vi "AO Repeat（Host）.vi"() -> ()   [LabVIEW 2019]
uses:
  <vilib>/FPGAPlugInAG/ELVIS III/niLvFpga_Open_ELVIS III.vi
  <vilib>/rvi/interface/common/dynamic/niFpgaDynamicAddResources.vi
  <vilib>/rvi/interface/common/niFpgaWaitOnOcc.vi
  <vilib>/Utility/error.llb/Error Cluster From Error Code.vi
  <vilib>/rvi/errors/niLvFpgaAdjustHostInterfaceError.vi
  <vilib>/FPGAPlugInAG/Dynamic/niLvFpga_Run_Dynamic.vi
  <vilib>/FPGAPlugInAG/Dynamic/niLvFpga_Abort_Dynamic.vi
  <vilib>/FPGAPlugInAG/Dynamic/niLvFpga_Close_Dynamic.vi
  <vilib>/rvi/interface/nirviOpenFPGA/nirviOpenFPGA.xnode
  FPGA Bitfiles/aiofpga_FPGATarget_AORepeat_+fFBwWQeRIY.lvbitx
  AO Repeat.vi
  <vilib>/rvi/interface/nirviMethod/nirviMethod.xnode
  <vilib>/rvi/interface/nirviReadWriteControl/nirviReadWriteControl.xnode
  <vilib>/rvi/interface/nirviCloseFPGA/nirviCloseFPGA.xnode
  <vilib>/FPGAPlugInAG/Dynamic/niLvFpga_ConfigureFifo_Dynamic.vi
  <vilib>/rvi/errors/niLvFpgaMergeErrorWithErrorCode.vi
  NiFpgaLv.dll
  <vilib>/rvi/interface/Simulation/niFpgaSimulationCallBeginRW.vi
  <vilib>/FPGAPlugInAG/Dynamic/niLvFpga_WriteFifo_Dynamic.vi
panel:
  in  "停止":bool
  in  "B1 采样率 [Hz] 4":dbl=10000.0 min=1000.0 max=1600000.0
  in  "B0 采样率 [Hz] 3":dbl=10000.0 min=1000.0 max=1600000.0
  in  "A1 采样率 [Hz] 2":dbl=10000.0 min=1000.0 max=1600000.0
  in  "A0 采样率 [Hz]":dbl=10000.0 min=1000.0 max=1600000.0
  in  "最大采样点数":dbl=10000.0
  in  "采样点数":u32=1000
  in  "B1 信号频率":dbl=400.0
  in  "B0 信号频率":dbl=200.0
  in  "A1 信号频率":dbl=100.0
  in  "A0 信号频率":dbl=10.0
  out "B1":dbl[](graph)
  out "B0":dbl[](graph)
  out "A1":dbl[](graph)
  out "A0":dbl[](graph)
  in  "Enable":bool[](array[boolean])=[TRUE, FALSE, TRUE, TRUE]
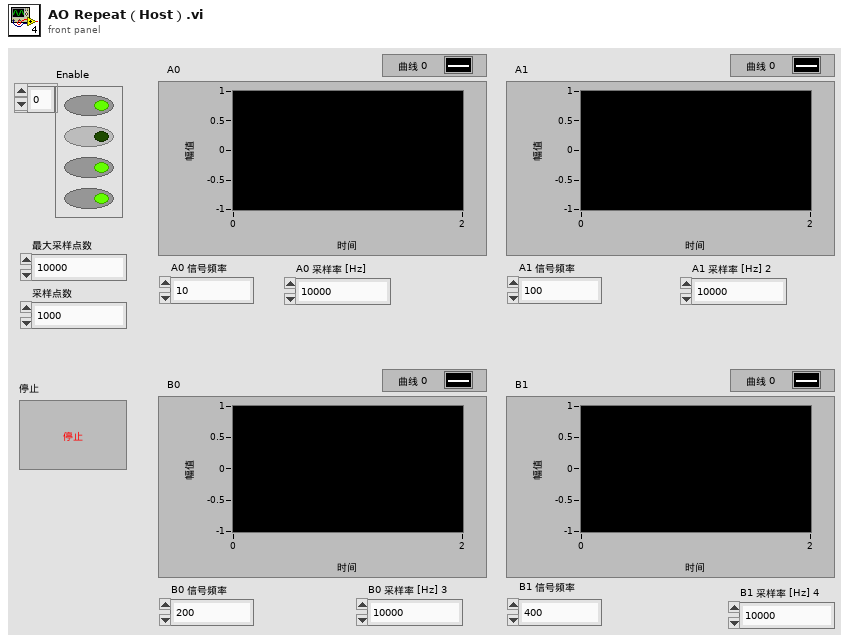
[diagram p1: front panel]
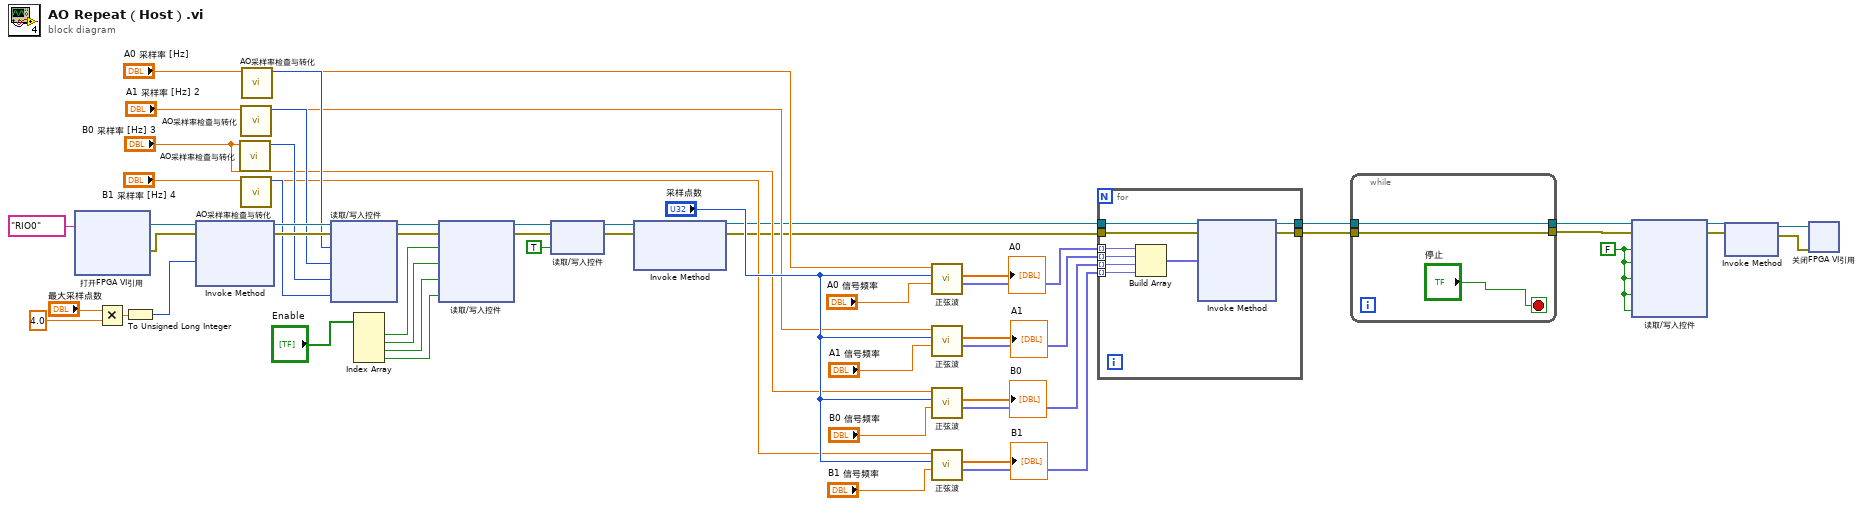
[diagram p0: block diagram]
diagram:
  w7 = FALSE ("开始")
  n1 = xnode "打开FPGA VI引用"("资源名称"=tag "RIO0") -> ("FPGA VI引用输出"=w51:refnum<k20>, "错误输出"=w52:errorcluster)  [unwired: 1 in]
  n2 = Multiply(x="最大采样点数", y=4.0) -> (x*y=w48:dbl)
  n3 = To Unsigned Long Integer(number=w48) -> (unsigned 32bit integer=w47:u32)
  n4 = xnode "Invoke Method"("FPGA VI引用输入"=w51, "错误输入"=w52, "请求的深度"=w47) -> ("FPGA VI引用输出"=w46:refnum<k20>, "错误输出"=w45:errorcluster)  [unwired: 1 out]
  n5 = call "AO采样率检查与转化.vi"("AO FIFO Sample Rate"="B0 采样率 [Hz] 3") -> ("Count (tick/s)"=w41:u32)  [unwired: 9 in, 1 out]
  n6 = call "AO采样率检查与转化.vi"("AO FIFO Sample Rate"="A1 采样率 [Hz] 2") -> ("Count (tick/s)"=w42:u32)  [unwired: 9 in, 1 out]
  n7 = call "AO采样率检查与转化.vi"("AO FIFO Sample Rate"="B1 采样率 [Hz] 4") -> ("Count (tick/s)"=w44:u32)  [unwired: 9 in, 1 out]
  n8 = call "AO采样率检查与转化.vi"("AO FIFO Sample Rate"="A0 采样率 [Hz]") -> ("Count (tick/s)"=w43:u32)  [unwired: 9 in, 1 out]
  n9 = xnode "读取/写入控件"("FPGA VI引用输入"=w46, "错误输入"=w45, "CNTRA0"=w43, "CNTRA1"=w42, "CNTRB0"=w41, "CNTRB1"=w44) -> ("FPGA VI引用输出"=w39:refnum<k20>, "错误输出"=w40:errorcluster)
  n10 = Index Array(array="Enable") -> (element #1=w37:bool, element #2=w36:bool, element #3=w35:bool, element #4=w34:bool)  [unwired: 4 in]
  n11 = xnode "读取/写入控件"("FPGA VI引用输入"=w39, "错误输入"=w40, "A0.Enable"=w37, "A1.Enable"=w36, "B0.Enable"=w35, "B1.Enable"=w34) -> ("FPGA VI引用输出"=w32:refnum<k20>, "错误输出"=w33:errorcluster)
  n12 = xnode "读取/写入控件"("FPGA VI引用输入"=w32, "错误输入"=w33, "开始"=TRUE) -> ("FPGA VI引用输出"=w29:refnum<k20>, "错误输出"=w30:errorcluster)
  n13 = xnode "Invoke Method"("FPGA VI引用输入"=w29, "错误输入"=w30) -> ("FPGA VI引用输出"=w14:refnum<k20>, "错误输出"=w15:errorcluster)  [unwired: 1 in]
  n14 = call "正弦波.vi"("信号频率 Hz"="A0 信号频率", "采样点数 S"="采样点数", "采样率 [Hz]"="A0 采样率 [Hz]") -> ("Sine 波形 FXP"=w19:fxp<+/-,20,5>[], "Sine 波形"=→"A0":dbl[])  [unwired: 7 in]
  n15 = call "正弦波.vi"("信号频率 Hz"="A1 信号频率", "采样点数 S"="采样点数", "采样率 [Hz]"="A1 采样率 [Hz] 2") -> ("Sine 波形 FXP"=w18:fxp<+/-,20,5>[], "Sine 波形"=→"A1":dbl[])  [unwired: 7 in]
  n16 = call "正弦波.vi"("信号频率 Hz"="B0 信号频率", "采样点数 S"="采样点数", "采样率 [Hz]"="B0 采样率 [Hz] 3") -> ("Sine 波形 FXP"=w17:fxp<+/-,20,5>[], "Sine 波形"=→"B0":dbl[])  [unwired: 7 in]
  n17 = call "正弦波.vi"("信号频率 Hz"="B1 信号频率", "采样点数 S"="采样点数", "采样率 [Hz]"="B1 采样率 [Hz] 4") -> ("Sine 波形 FXP"=w16:fxp<+/-,20,5>[], "Sine 波形"=→"B1":dbl[])  [unwired: 7 in]
  n18 = for {
    tunnel: w19 -> [w62] mode=indexing
    tunnel: w18 -> [w61] mode=indexing
    tunnel: w17 -> [w60] mode=indexing
    tunnel: w16 -> [w59] mode=indexing
    tunnel: w14 -> [w58]
    tunnel: w15 -> [w57]
    tunnel: [w55] -> w9
    tunnel: [w54] -> w8
    n19 = Build Array(w62, w61, w60, w59) -> (w56:fxp<+/-,20,5>[])
    n20 = xnode "Invoke Method"("FPGA VI引用输入"=w58, "错误输入"=w57, "数据"=w56) -> ("FPGA VI引用输出"=w54:refnum<k20>, "错误输出"=w55:errorcluster)  [unwired: 1 in, 1 out]
  }
  n21 = while {
    tunnel: [w64] -> w2
    tunnel: w9 -> [w64]
    tunnel: w8 -> [w63]
    tunnel: [w63] -> w1
    stop <- "停止" stop-if-true
  }
  n22 = xnode "读取/写入控件"("FPGA VI引用输入"=w1, "错误输入"=w2, "开始"=w7, "A0.Enable"=w7, "A1.Enable"=w7, "B0.Enable"=w7, "B1.Enable"=w7) -> ("FPGA VI引用输出"=w5:refnum<k20>, "错误输出"=w6:errorcluster)
  n23 = xnode "Invoke Method"("FPGA VI引用输入"=w5, "错误输入"=w6) -> ("FPGA VI引用输出"=w3:refnum<k20>, "错误输出"=w4:errorcluster)
  n24 = xnode "关闭FPGA VI引用"("FPGA VI引用输入"=w3, "错误输入"=w4) -> ()  [unwired: 1 out]
